vi "BenchA_v09_97.vi"() -> ()   [LabVIEW 2017]
uses:
  x64/Debug/BERTTA.dll
panel:
  out "element":bool
  out "Started:":string
  in  "SHUTDOWN":bool
  in  "MASTER CONTROL":bool
  in  "Tab Control":T1(tab)
  out "Output File":path caption="selected path"
  in  "Browse folder":path=path "" caption="start path"
  in  "Read Seq":bool
  in  "Save Seq":bool
  in  "Configuration file":path=path "C:/Users/shresplab/Desktop/BerttaConfiguration.lvm" caption="Filename"
  in  "OK Button 2":bool
  out "Boolean":bool
  in  "User (initials)":string
  in  "Project name":string
  in  "Description":string
  out "PUMP1":bool
  out "Target amount":dbl
  out "Scale weight":dbl
  out "Amount now":dbl
  out "Flow rate":dbl
  out "Time to target":dbl format="%<%H:%M:%S>t"
  out "Current step":dbl
  out "Target":dbl
  out "Amount now":dbl
  out "Amount now":dbl
  out "Target":dbl
  out "Current step":dbl
  out "Time to target":dbl format="%<%H:%M:%S>t"
  out "Flow rate":dbl
  out "Amount now":dbl
  out "Scale weight":dbl
  out "Target amount":dbl
  out "PUMP2":bool
  out "Sensor OK 6":bool
  out "Sensor OK 5":bool
  out "Sensor OK 4":bool
  out "Sensor OK 3":bool
  in  "OK Button":bool
  in  "Add comment":string
  out "PUMP3":bool
  out "Target amount":dbl
  out "Scale weight":dbl
  out "Amount now":dbl
  out "Flow rate":dbl
  out "Time to target":dbl format="%<%H:%M:%S>t"
  out "Current step":dbl
  out "Target":dbl
  out "Amount now":dbl
  out "Tr":dbl
  out "Tj in":dbl
  out "Tj out":dbl
  out "T set":dbl
  out "Current step":i32
  out "RPM":dbl
  out "Torque 2":dbl
  out "Waveform Chart 5":dynamicdata(graph)
  out "Waveform Chart 6":dynamicdata(graph)
  out "Waveform Chart 7":dynamicdata(graph)
  in  "Tab Control 2":T2(tab)
  out "Waveform Chart 3":dynamicdata(graph)
  out "Waveform Chart 8":dynamicdata(graph)
  out "Waveform Chart 11":dynamicdata(graph)
  out "Waveform Chart 13":dynamicdata(graph)
  out "Waveform Chart 9":dynamicdata(graph)
  out "Table":string[][](table)=[["14.8.2017 18.06.59", "0,000000", "417,670000", "-0,150000", "1,000000", "22,220000", "23,366837", "23,574959", "23,985852", "23,690000", "240,000000", "4,000000", "0,000000", "397,000000", "-397,000000", "1,000000"], ["14.8.2017 18.07.06", "0,000000", "417,640000", "-0,120000", "1,000000", "22,220000", "23,763115", "23,906257", "23,985694", "23,680000", "240,000000", "4,000000", "0,000000", "397,000000", "-397,000000", "1,000000"], ["14.8.2017 18.07.13", "0,000000", "417,640000", "-0,120000", "1,000000", "22,220000", "23,965922", "24,013440", "23,984906", "23,670000", "240,000000", "4,100000", "3,000000", "397,000000", "-397,000000", "1,000000"], ["14.8.2017 18.07.21", "0,000000", "417,640000", "-0,120000", "1,000000", "22,220000", "23,943860", "23,900110", "23,987113", "23,670000", "240,000000", "4,000000", "0,000000", "397,000000", "-397,000000", "1,000000"], ["14.8.2017 18.07.28", "0,000000", "417,640000", "-0,120000", "1,000000", "22,220000", "23,736328", "23,600018", "23,989004", "23,660000", "240,000000", "4,000000", "0,000000", "397,000000", "-397,000000", "1,000000"], ["14.8.2017 18.07.36", "0,000000", "417,640000", "-0,120000", "1,000000", "22,220000", "23,480910", "23,324538", "23,991053", "23,660000", "240,000000", "4,000000", "0,000000", "397,000000", "-397,000000", "1,000000"], ["14.8.2017 18.07.43", "0,000000", "417,640000", "-0,120000", "2,000000", "22,220000", "23,195579", "23,008270", "23,999093", "23,650000", "240,000000", "4,000000", "0,000000", "397,000000", "-397,000000", "1,000000"], ["14.8.2017 18.07.51", "0,000000", "417,650000", "-417,650000", "1,000000", "22,220000", "22,862541", "22,649021", "24,003979", "23,650000", "240,000000", "4,000000", "0,000000", "397,000000", "-397,000000", "2,000000"], ["14.8.2017 18.07.58", "0,000000", "417,640000", "0,010000", "1,000000", "22,220000", "22,541353", "22,354878", "24,005398", "23,650000", "240,000000", "4,000000", "0,000000", "397,000000", "-397,000000", "1,000000"], ["14.8.2017 18.08.06", "0,000000", "417,640000", "0,010000", "1,000000", "22,220000", "22,347931", "22,253738", "24,007605", "23,640000", "240,000000", "4,100000", "0,000000", "397,000000", "-397,000000", "1,000000"], ["14.8.2017 18.08.13", "0,000000", "417,640000", "0,010000", "1,000000", "22,220000", "22,329030", "22,302102", "24,006028", "23,640000", "240,000000", "4,000000", "0,000000", "395,820000", "-395,820000", "1,000000"], ["14.8.2017 18.08.20", "0,000000", "417,640000", "0,010000", "1,000000", "22,220000", "22,466849", "22,511320", "24,002403", "23,630000", "240,000000", "4,000000", "0,000000", "395,830000", "-0,010000", "1,000000"], ["14.8.2017 18.08.28", "0,000000", "417,640000", "0,010000", "1,000000", "22,220000", "22,707062", "22,835101", "24,000984", "23,620000", "240,000000", "4,000000", "0,000000", "395,830000", "-0,010000", "1,000000"], ["14.8.2017 18.08.35", "0,000000", "417,640000", "0,010000", "1,000000", "22,220000", "23,054104", "23,232979", "24,001299", "23,600000", "240,000000", "4,000000", "0,000000", "395,830000", "-0,010000", "1,000000"], ["14.8.2017 18.08.43", "0,000000", "417,640000", "0,010000", "1,000000", "22,220000", "23,412371", "23,522793", "24,002560", "23,590000", "240,000000", "4,000000", "0,000000", "395,820000", "0,000000", "1,000000"], ["14.8.2017 18.08.51", "0,000000", "417,640000", "0,010000", "1,000000", "22,220000", "23,596247", "23,656125", "24,003821", "23,580000", "240,000000", "4,000000", "0,000000", "395,820000", "0,000000", "1,000000"]]
  out "Boolean 4":bool
  out "Boolean 3":bool
  out "Boolean 2":bool
  in  "Reset 6":bool
  in  "Manual/Ramp":bool=TRUE
  in  "Array":dbl[][](array[numeric])=[[20.0, 0.0], [20.0, 0.0], [20.0, 0.0]]
  in  "?":bool
  in  "Time":dbl format="Time to target (min):                %#_g"
  out "Current temp":dbl format="Current temperature (S1):   %#_6g"
  in  "OK Button 3":bool
  in  "T ext / T ext 2":enum32{"Sensor 1", "Sensor 2"}(radio)
  out "Sensor OK":bool
  in  "T fail":dbl=20.0 format="Failsafe temperature:              %#_g"
  in  "Setpoint":dbl=20.0 format="Temperature target:                %#_6g"
  in  "Manual select":T3(radio)
  out "Waveform Chart":dynamicdata(graph)
  out "T external 2":dbl format="Current temperature (S2):    %#_g"
  in  "UPDATE TEMP":bool
  out "Led11 5":bool
  out "RPM":dbl format="%_4f"
  out "Led10 3":bool
  out "Led9 3":bool
  out "Led8 3":bool
  out "Led7 3":bool
  out "Led6 3":bool
  out "Led5 3":bool
  out "Led4 3":bool
  out "Led3 3":bool
  out "Led2 3":bool
  out "Led1 3":bool
  in  "PumpSeq 4":dbl[][](array[numeric])=[[0.0, 0.0, 0.0, 0.0, 0.0, 0.0, 0.0, 0.0, 0.0, 0.0], [0.0, 0.0, 0.0, 0.0, 0.0, 0.0, 0.0, 0.0, 0.0, 0.0], [0.0, 0.0, 0.0, 0.0, 0.0, 0.0, 0.0, 0.0, 0.0, 0.0], [0.0, 0.0, 0.0, 0.0, 0.0, 0.0, 0.0, 0.0, 0.0, 0.0], [0.0, 0.0, 0.0, 0.0, 0.0, 0.0, 0.0, 0.0, 0.0, 0.0], [0.0, 0.0, 0.0, 0.0, 0.0, 0.0, 0.0, 0.0, 0.0, 0.0], [0.0, 0.0, 0.0, 0.0, 0.0, 0.0, 0.0, 0.0, 0.0, 0.0], [0.0, 0.0, 0.0, 0.0, 0.0, 0.0, 0.0, 0.0, 0.0, 0.0], [0.0, 0.0, 0.0, 0.0, 0.0, 0.0, 0.0, 0.0, 0.0, 0.0], [0.0, 0.0, 0.0, 0.0, 0.0, 0.0, 0.0, 0.0, 0.0, 0.0]]
  in  "?":bool
  out "Flow rate (g/min)":dbl
  out "Scale reading":dbl
  out "Step amount now":dbl
  in  "Grams / min":dbl
  out "Waveform Chart 14":dynamicdata(graph)
  in  "?":bool
  out "Total amount now":dbl
  out "Led11 4":bool
  in  "Reset 5":bool
  out "Elapsed / step":i32
  out "Time to target":dbl format="%<%H:%M:%S>t"
  in  "OK Button 4":bool
  out "Led11":bool
  out "RPM":dbl format="%_4f"
  out "Led10":bool
  out "Led9":bool
  out "Led8":bool
  out "Led7":bool
  out "Led6":bool
  out "Led5":bool
  out "Led4":bool
  out "Led3":bool
  out "Led2":bool
  out "Led1":bool
  in  "PumpSeq 2":dbl[][](array[numeric])=[[0.0, 0.0, 0.0, 0.0, 0.0, 0.0, 0.0, 0.0, 0.0, 0.0], [0.0, 0.0, 0.0, 0.0, 0.0, 0.0, 0.0, 0.0, 0.0, 0.0], [0.0, 0.0, 0.0, 0.0, 0.0, 0.0, 0.0, 0.0, 0.0, 0.0], [0.0, 0.0, 0.0, 0.0, 0.0, 0.0, 0.0, 0.0, 0.0, 0.0], [0.0, 0.0, 0.0, 0.0, 0.0, 0.0, 0.0, 0.0, 0.0, 0.0], [0.0, 0.0, 0.0, 0.0, 0.0, 0.0, 0.0, 0.0, 0.0, 0.0], [0.0, 0.0, 0.0, 0.0, 0.0, 0.0, 0.0, 0.0, 0.0, 0.0], [0.0, 0.0, 0.0, 0.0, 0.0, 0.0, 0.0, 0.0, 0.0, 0.0], [0.0, 0.0, 0.0, 0.0, 0.0, 0.0, 0.0, 0.0, 0.0, 0.0], [0.0, 0.0, 0.0, 0.0, 0.0, 0.0, 0.0, 0.0, 0.0, 0.0]]
  in  "?":bool
  out "Flow rate (g/min)":dbl
  out "Scale reading":dbl
  out "Step amount now":dbl
  in  "Grams / min":dbl
  out "Waveform Chart 10":dynamicdata(graph)
  in  "?":bool
  out "Total amount now":dbl
  out "Led11":bool
  in  "Reset 3":bool
  out "Elapsed / step":i32
  out "Time to target":dbl format="%<%H:%M:%S>t"
  in  "OK Button 5":bool
  out "Led11 3":bool
  out "RPM":dbl format="%_4f"
  out "Led10 2":bool
  out "Led9 2":bool
  out "Led8 2":bool
  out "Led7 2":bool
  out "Led6 2":bool
  out "Led5 2":bool
  out "Led4 2":bool
  out "Led3 2":bool
  out "Led2 2":bool
  out "Led1 2":bool
  in  "PumpSeq 3":dbl[][](array[numeric])=[[0.0, 0.0, 0.0, 0.0, 0.0, 0.0, 0.0, 0.0, 0.0, 0.0], [0.0, 0.0, 0.0, 0.0, 0.0, 0.0, 0.0, 0.0, 0.0, 0.0], [0.0, 0.0, 0.0, 0.0, 0.0, 0.0, 0.0, 0.0, 0.0, 0.0], [0.0, 0.0, 0.0, 0.0, 0.0, 0.0, 0.0, 0.0, 0.0, 0.0], [0.0, 0.0, 0.0, 0.0, 0.0, 0.0, 0.0, 0.0, 0.0, 0.0], [0.0, 0.0, 0.0, 0.0, 0.0, 0.0, 0.0, 0.0, 0.0, 0.0], [0.0, 0.0, 0.0, 0.0, 0.0, 0.0, 0.0, 0.0, 0.0, 0.0], [0.0, 0.0, 0.0, 0.0, 0.0, 0.0, 0.0, 0.0, 0.0, 0.0], [0.0, 0.0, 0.0, 0.0, 0.0, 0.0, 0.0, 0.0, 0.0, 0.0], [0.0, 0.0, 0.0, 0.0, 0.0, 0.0, 0.0, 0.0, 0.0, 0.0]]
  in  "?":bool
  out "Flow rate (g/min)":dbl
  out "Scale reading":dbl
  out "Step amount now":dbl
  in  "Grams / min":dbl
  out "Waveform Chart 12":dynamicdata(graph)
  in  "?":bool
  out "Total amount now":dbl
  out "Led11 2":bool
  in  "Reset 4":bool
  out "Elapsed / step":i32
  out "Time to target":dbl format="%<%H:%M:%S>t"
  in  "OK Button 6":bool
  in  "Remote / Manual":bool
  in  "Set RPM":i32
  out "RPM":dbl
  out "Torque":dbl
  out "Waveform Chart 4":dynamicdata(graph)
  in  "OK Button 7":bool
  out "PortDev out":dbl[](array[numeric])
  in  "Save PortDev":bool
  out "PortDev in":dbl[](array[numeric])
  in  "dev1":i32
  in  "dev2":i32
  in  "dev3":i32
  in  "dev4":i32
  in  "dev5":i32
  in  "dev6":i32
  in  "dev8":i32
  in  "port1":i32
  in  "port2":i32
  in  "port3":i32
  in  "port4":i32
  in  "port5":i32
  in  "port6":i32
  in  "port7":i32
  in  "port8":i32
  in  "dev7":i32
  in  "Treshold (T/C)":dbl=0.5
  out "DAQ 9217 (PT100)":errorcluster
  out "Config File":dbl[][](array[numeric])
  # "Temperature sensor:"
  # "Manual control:"
  # "PUMP & SCALE 1"
  # "STEP"
  # "TOTAL"
  # "PUMP & SCALE 2"
  # "STEP"
  # "TOTAL"
  # "PUMP & SCALE 3"
  # "STEP"
  # "TOTAL"
  # "Temperature control parameter"
  # "Secondary temperature sensor"
  # "Temp target"
  # "Time target"
  # "Grams    /   min"
  # "End of sequence"
  # "Manual control"
  # "Grams    /   min"
  # "End of sequence"
  # "Manual control"
  # "Grams    /   min"
  # "End of sequence"
  # "Manual control"
  # "dev1 and dev2 always to port1 and 2\nport1 = port2 = Lauda\n\ndev3 and dev4 always to port3 and port4\nport3 = port4 = Heidolph"
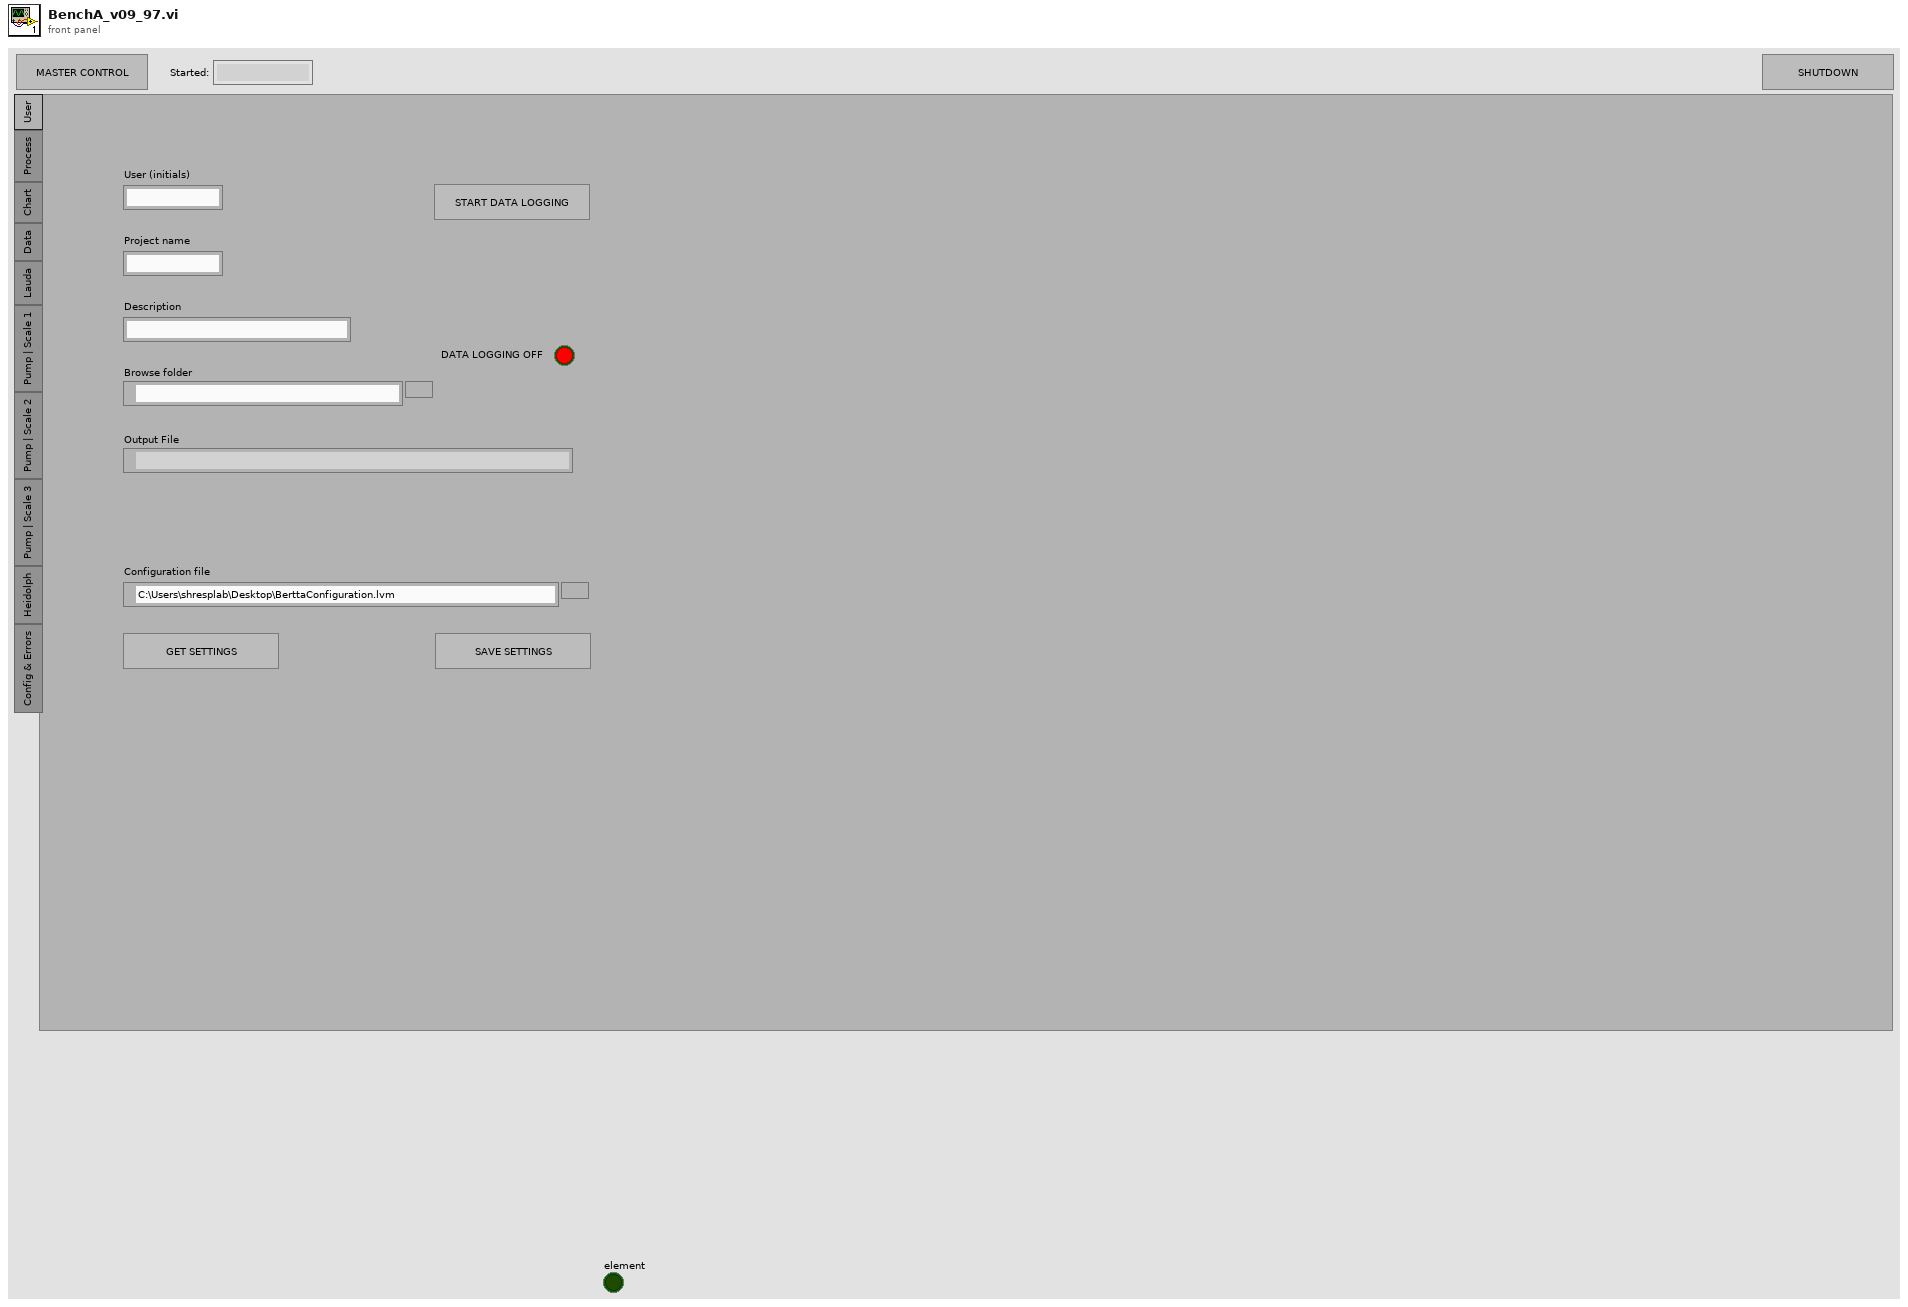
[diagram p1: front panel]
types:
  T1 = enum32{"User", "Process", "Chart", "Data", "Lauda", "Pump | Scale 1", "Pump | Scale 2", "Pump | Scale 3", "Heidolph", "Config & Errors"}
  T2 = enum32{"Temperatures", "Scale / Pump 1", "Scale / Pump 2", "Scale / Pump 3", "RPM / torque"}
  T3 = enum32{"Reactor temperature", "Jacket temperature"}
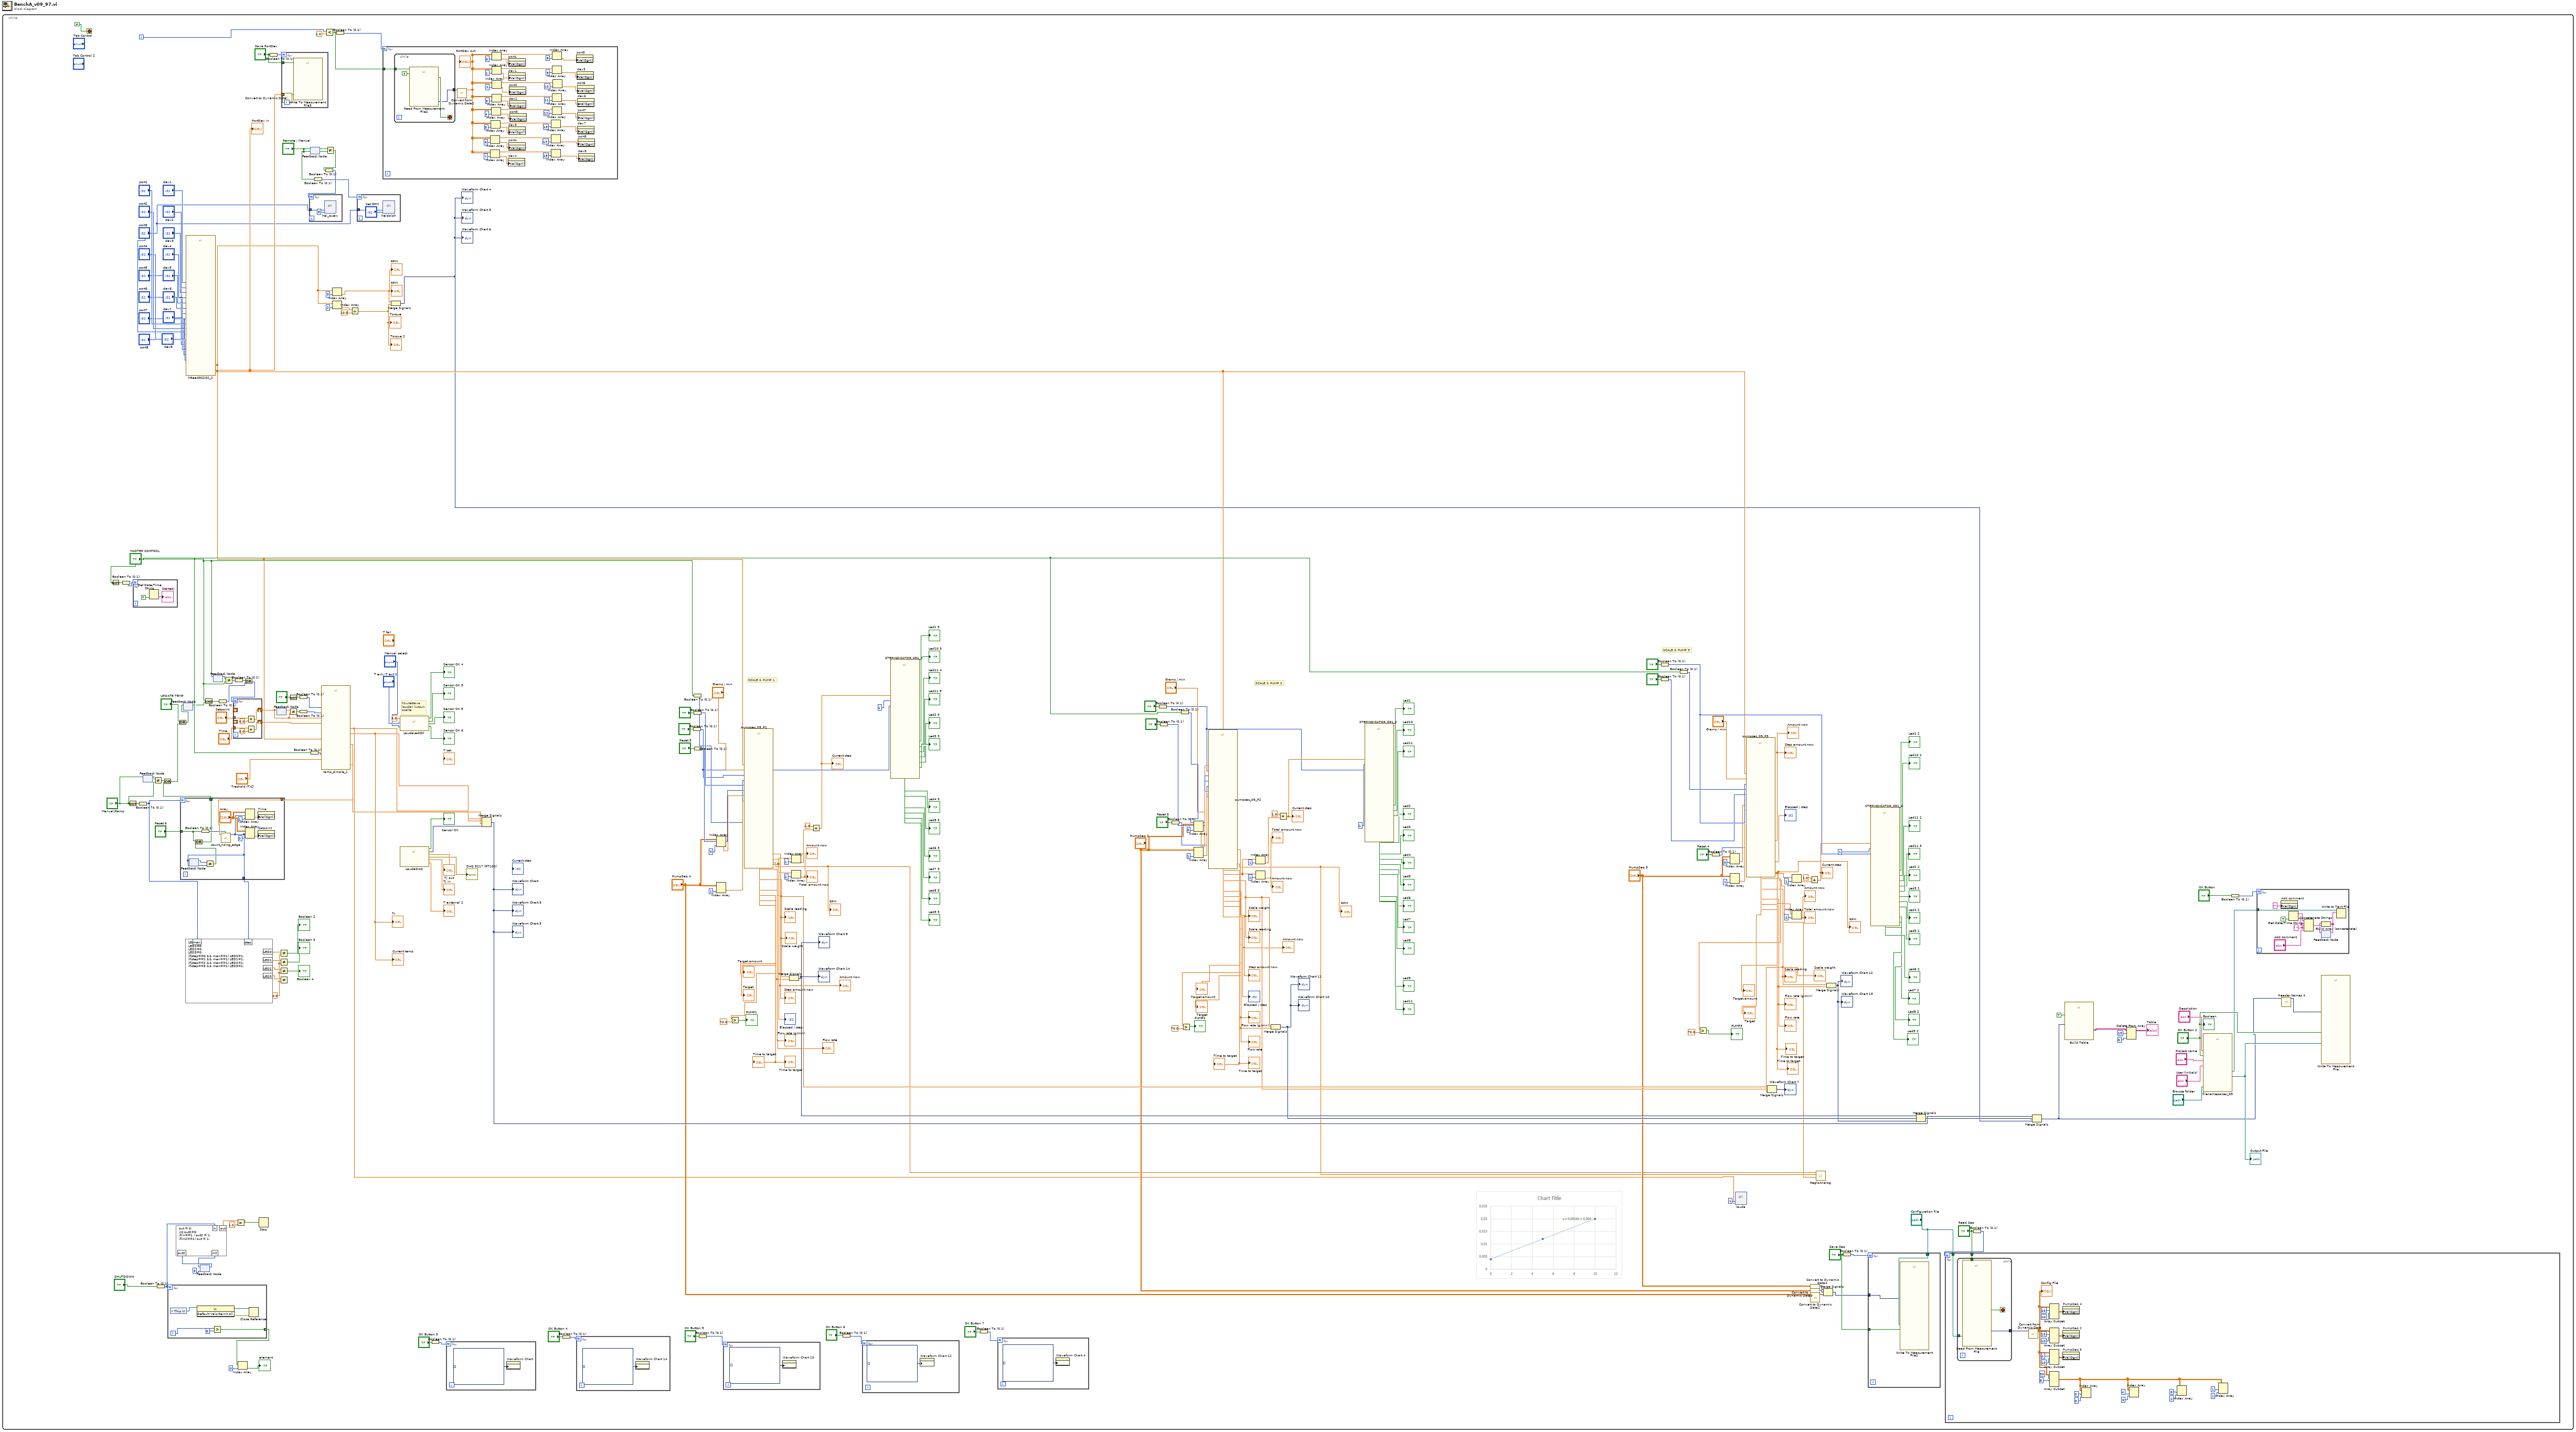
[diagram p0: block diagram]
diagram:
  n1 = while {
    i -> [w47]
    stop <- FALSE stop-if-true
    w33 = 0.0 ("y")
    # "Muutettava\nlaudan kutsun \nosalta"
    # "SCALE & PUMP 1"
    # "SCALE & PUMP 3"
    # "SCALE & PUMP 2"
    n2 = Not(x="MASTER CONTROL") -> (.not. x?=w275:bool)
    n3 = Boolean To (0,1)(Boolean=w275) -> (0, 1=w276:i16)
    n4 = Not(x="Manual/Ramp") -> (.not. x?=w40:bool)
    n5 = for {
      N: w276 -> [_]
      n6 = Get Date/Time String(want seconds? (F)=TRUE) -> (time string=→"Started:":string)  [unwired: 2 in, 1 out]
    }
    n7 = Boolean To (0,1)(Boolean=w40) -> (0, 1=w22:i16)
    n8 = feedback #1() -> (w28:bool)  [unwired: 1 in]
    n9 = feedback-in #1("Manual/Ramp") -> ()
    n10 = Not Equal?(x=w28, y="Manual/Ramp") -> (x != y?=w25:bool)
    n11 = Boolean To (0,1)(Boolean="SHUTDOWN") -> (0, 1=w260:i16)
    n12 = for {
      N: w260 -> [_]
      tunnel: [w391] -> w274 mode=indexing
      i -> [w393]
      n13 = control-ref of="This VI"() -> (w396:refnum<vi>)
      n14 = invoke class="VI" method="Default Vals.Reinit All"(reference=w396) -> (reference out=w394:refnum<vi>, error out=w395:errorcluster)  [unwired: 2 in, 1 out]
      n15 = Greater?(x=w393, y=0) -> (0:w391:bool)
      n16 = Close Reference(reference=w394, error in (no error)=w395) -> ()  [unwired: 1 out]
    }
    n17 = feedback #2() -> (w20:bool)  [unwired: 1 in]
    n18 = call "MReadRS232_2.vi"("port1"="port1", "dev1"="dev1", "port2"="port2", "dev2"="dev2", "port3"="port3", "dev7"="dev7", "dev8"="dev8", "port7"="port7", "port8"="port8", "dev5"="dev5", "port5"="port5", "dev4"="dev4", "dev6"="dev6", "port6"="port6", "port4"="port4", "dev3"="dev3") -> ("output array"=w51:dbl[], "params"=w12:dbl[])  [unwired: 2 in]
    "PortDev in" <- w51
    n19 = feedback #3(0) -> (w258:i32)
    n20 = formula code="out = 0;\nint out2=0;\nif(in==1 ) out2 = 1;\nif(in2==1) out = 1;"("in"=w260, "in2"=w258) -> ("out"=w262:dbl, "out2"=w259:i32)
    n21 = feedback-in #3(w259) -> ()
    n22 = And(x="MASTER CONTROL", y=w20) -> (x .and. y?=w80:bool)
    n23 = feedback #4() -> (w71:bool)  [unwired: 1 in]
    n24 = feedback-in #4("MASTER CONTROL") -> ()
    n25 = Boolean To (0,1)(Boolean=w80) -> (0, 1=w68:i16)
    n26 = Not Equal?(x=w71, y="MASTER CONTROL") -> (x != y?=w70:bool)
    n27 = Boolean To (0,1)(Boolean=w70) -> (0, 1=w67:i16)
    n28 = Equal?(x=w262, y=1.0) -> (x = y?=w261:bool)
    n29 = Index Array(array=w274, index=0) -> (element=→"element":bool)
    n30 = Or(x=w67, y=w68) -> (x .or. y?=w66:i16)
    n31 = for {
      N: w66 -> [_]
      tunnel: "Time" -> [w343]
      shift-right: [w342] -> w81
      shift-left: _ -> [_]
      tunnel: "Setpoint" -> [w340]
      shift-right: [w339] -> w78
      shift-left: _ -> [_]
      n32 = Add(x=w340, y=0.0) -> (x+y=w339:dbl)
      n33 = Add(x=w343, y=0.0) -> (x+y=w342:dbl)
    }
    n34 = Stop(stop? (T)=w261) -> ()
    n35 = Boolean To (0,1)(Boolean="Save PortDev") -> (0, 1=w50:i16)
    n36 = feedback-in #5(w78) -> ()
    n37 = feedback #5() -> (w79:dbl)  [unwired: 1 in]
    n38 = for {
      N: w50 -> [_]
      tunnel: w51 -> [w338]
      tunnel: "Save PortDev" -> [w336]
      n39 = call "Convert to Dynamic Data"("Array"=w338) -> ("Dynamic Data Type"=w337:dynamicdata)  [unwired: 3 in]
      n40 = call "Write To Measurement File3"("Signals"=w337, "Reset"=w336) -> ()  [unwired: 15 in, 3 out]
    }
    n41 = Not(x="?") -> (.not. x?=w74:bool)
    n42 = Not Equal?(x=w79, y=w78) -> (x != y?=w77:bool)
    n43 = Boolean To (0,1)(Boolean=w74) -> (0, 1=w76:i16)
    n44 = Boolean To (0,1)(Boolean=w77) -> (0, 1=w72:i16)
    n45 = Boolean To (0,1)(Boolean="MASTER CONTROL") -> (0, 1=w73:i16)
    n46 = feedback-in #6("Remote / Manual") -> ()
    n47 = feedback #6() -> (w17:bool)  [unwired: 1 in]
    n48 = Boolean To (0,1)(Boolean="Remote / Manual") -> (0, 1=w15:i16)
    n49 = call "ramp_simple_1.vi"("array"=w12, "treshold"="Treshold (T/C)", "time_set"=w81, "T_sp"=w78, "master"=w73, "reset"=w72, "pause"=w76) -> ("T control"=w1:dbl, "Tr"=w85:dbl, "Tin"=w84:dbl, "target_reached"=w38:dbl)  [unwired: 1 out]
    "Tr" <- w85
    "Current temp" <- w85
    n50 = for {
      N: w22 -> [_]
      tunnel: w38 -> [w295]
      tunnel: [w285] -> w26
      tunnel: "Reset 6" -> [w287]
      tunnel: [w288] -> w29
      n51 = feedback #7() -> (w289:i32)  [unwired: 1 in]
      n52 = Boolean To (0,1)(Boolean=w287) -> (0, 1=w290:i16)
      n53 = call "count_rising_edge.vi"("reset"=w290, "target_reached"=w295) -> ("element 2"=w288:i32)  [unwired: 9 in]
      n54 = feedback-in #7(w288) -> ()
      n55 = Not Equal?(x=w289, y=w288) -> (x != y?=w286:bool)
      n56 = Or(x=w287, y=w286) -> (x .or. y?=w285:bool)
      n57 = Index Array(array="Array", index (row)=w288, index (col)=1 ("disabled index (col)")) -> (element=w291:dbl)
      n58 = Index Array(array="Array", index (row)=w288, index (col)=0 ("disabled index (col)")) -> (element=w292:dbl)
      n59 = property on="Time" class="DigNum (strict)"("Val(Sgnl)"=w291) -> ()  [unwired: 2 in, 2 out]
      n60 = property on="Setpoint" class="DigNum (strict)"("Val(Sgnl)"=w292) -> ()  [unwired: 2 in, 2 out]
    }
    n61 = Or(x=w25, y=w26) -> (x .or. y?=w24:bool)
    n62 = Or(x="UPDATE TEMP", y=w24) -> (x .or. y?=w21:bool)
    n63 = feedback-in #2(w21) -> ()
    n64 = formula code="LED0=0;\nLED1=0;\nLED2=0;\nLED3=0;\nif(step==0 && man==1) LED0=1;\nif(step==1 && man==1) LED1=1;\nif(step==2 && man==1) LED2=1;\nif(step==3 && man==1) LED3=1;"("step"=w29, "man"=w22) -> ("LED0"=w37:dbl, "LED1"=w36:dbl, "LED2"=w35:dbl, "LED3"=w34:dbl)
    n65 = Not Equal?(x=w37, y=w33) -> (x != y?=→"Boolean 2":bool)
    n66 = Not Equal?(x=w36, y=w33) -> (x != y?=→"Boolean 3":bool)
    n67 = Not Equal?(x=w35, y=w33) -> (x != y?=→"Boolean 4":bool)
    n68 = Not Equal?(x=w34, y=w33) -> ()  [unwired: 1 out]
    n69 = Less?(x=w47, y=1.0) -> (x < y?=w45:bool)
    n70 = Not Equal?(x=w17, y="Remote / Manual") -> (x != y?=w16:bool)
    n71 = Boolean To (0,1)(Boolean=w16) -> (0, 1=w18:i16)
    n72 = for {
      N: w18 -> [_]
      tunnel: "port3" -> [w283]
      n73 = dll-call lib="C:/Users/shresplab/OneDrive - Kemira Oyj/Documents/GitHub/Bertta/BERTTA/x64/Debug/BERTTA.dll" fn="hei_query"("port"=w283, "q"=5) -> ()  [unwired: 6 in, 2 out]
    }
    n74 = Index Array(array=w12, index=3) -> (element=w9:dbl)
    "RPM" <- w9
    "RPM" <- w9
    n75 = Index Array(array=w12, index=2) -> (element=w11:dbl)
    n76 = Boolean To (0,1)(Boolean=w45) -> (0, 1=w46:i16)
    n77 = Divide(x=w11, y=10.0) -> (x/y=w8:dbl)
    "Torque" <- w8
    "Torque 2" <- w8
    n78 = for {
      N: w15 -> [_]
      tunnel: "port3" -> [w281]
      n79 = dll-call lib="C:/Users/shresplab/OneDrive - Kemira Oyj/Documents/GitHub/Bertta/BERTTA/x64/Debug/BERTTA.dll" fn="heidolph"("port"=w281, "speed"="Set RPM") -> ()  [unwired: 6 in, 2 out]
    }
    n80 = for {
      N: w46 -> [_]
      tunnel: w45 -> [w331]
      n81 = while {
        tunnel: [w334] -> w330
        tunnel: w331 -> [w332]
        stop <- w335 stop-if-true
        n82 = call "Read From Measurement File2"("Enable"=TRUE, "Reset"=w332) -> ("Signals"=w334:dynamicdata, "EOF?"=w335:bool)  [unwired: 4 in, 4 out]
      }
      n83 = call "Convert from Dynamic Data2"("Dynamic Data Type"=w330) -> ("Array"=w313:dbl[])  [unwired: 3 in]
      "PortDev out" <- w313
      n84 = Index Array(array=w313, index=6) -> (element=w306:dbl)
      n85 = Index Array(array=w313, index=7) -> (element=w305:dbl)
      n86 = Index Array(array=w313, index=5) -> (element=w307:dbl)
      n87 = Index Array(array=w313, index=4) -> (element=w308:dbl)
      n88 = Index Array(array=w313, index=0) -> (element=w312:dbl)
      n89 = Index Array(array=w313, index=1) -> (element=w311:dbl)
      n90 = Index Array(array=w313, index=3) -> (element=w309:dbl)
      n91 = Index Array(array=w313, index=2) -> (element=w310:dbl)
      n92 = property on="dev4" class="DigNum (strict)"("Val(Sgnl)"=w305) -> ()  [unwired: 2 in, 2 out]
      n93 = property on="dev3" class="DigNum (strict)"("Val(Sgnl)"=w307) -> ()  [unwired: 2 in, 2 out]
      n94 = property on="port4" class="DigNum (strict)"("Val(Sgnl)"=w306) -> ()  [unwired: 2 in, 2 out]
      n95 = property on="port1" class="DigNum (strict)"("Val(Sgnl)"=w312) -> ()  [unwired: 2 in, 2 out]
      n96 = property on="dev1" class="DigNum (strict)"("Val(Sgnl)"=w311) -> ()  [unwired: 2 in, 2 out]
      n97 = property on="port2" class="DigNum (strict)"("Val(Sgnl)"=w310) -> ()  [unwired: 2 in, 2 out]
      n98 = property on="dev2" class="DigNum (strict)"("Val(Sgnl)"=w309) -> ()  [unwired: 2 in, 2 out]
      n99 = property on="port3" class="DigNum (strict)"("Val(Sgnl)"=w308) -> ()  [unwired: 2 in, 2 out]
      n100 = Index Array(array=w313, index=14) -> (element=w298:dbl)
      n101 = Index Array(array=w313, index=15) -> (element=w297:dbl)
      n102 = Index Array(array=w313, index=13) -> (element=w299:dbl)
      n103 = Index Array(array=w313, index=12) -> (element=w300:dbl)
      n104 = Index Array(array=w313, index=8) -> (element=w304:dbl)
      n105 = Index Array(array=w313, index=9) -> (element=w303:dbl)
      n106 = Index Array(array=w313, index=11) -> (element=w301:dbl)
      n107 = Index Array(array=w313, index=10) -> (element=w302:dbl)
      n108 = property on="port5" class="DigNum (strict)"("Val(Sgnl)"=w304) -> ()  [unwired: 2 in, 2 out]
      n109 = property on="dev5" class="DigNum (strict)"("Val(Sgnl)"=w303) -> ()  [unwired: 2 in, 2 out]
      n110 = property on="port6" class="DigNum (strict)"("Val(Sgnl)"=w302) -> ()  [unwired: 2 in, 2 out]
      n111 = property on="dev6" class="DigNum (strict)"("Val(Sgnl)"=w301) -> ()  [unwired: 2 in, 2 out]
      n112 = property on="port7" class="DigNum (strict)"("Val(Sgnl)"=w300) -> ()  [unwired: 2 in, 2 out]
      n113 = property on="dev7" class="DigNum (strict)"("Val(Sgnl)"=w299) -> ()  [unwired: 2 in, 2 out]
      n114 = property on="port8" class="DigNum (strict)"("Val(Sgnl)"=w298) -> ()  [unwired: 2 in, 2 out]
      n115 = property on="dev8" class="DigNum (strict)"("Val(Sgnl)"=w297) -> ()  [unwired: 2 in, 2 out]
    }
    n116 = Merge Signals(w9, w8) -> (w7:dynamicdata)
    "Waveform Chart 4" <- w7
    "Waveform Chart 6" <- w7
    "Waveform Chart 9" <- w7
    n117 = call "LaudaLedCtrl.vi"("Manual select"="Manual select", "T ext / T ext in"="T ext / T ext 2", "Lauda port"=9.0) -> ("Sensor OK 5"=→"Sensor OK 5":bool, "Sensor OK 3"=→"Sensor OK 3":bool, "Sensor OK 4"=→"Sensor OK 4":bool, "Sensor OK 6"=→"Sensor OK 6":bool)  [unwired: 5 in]
    n118 = call "LaudaDAQ.vi"() -> ("error out"=→"DAQ 9217 (PT100)":errorcluster, 1:"Tj out"=→"Tj out":dbl, "data"=w150:dynamicdata, "Sensor OK"=→"Sensor OK":bool, 4:"Tj out"=→"Tj in":dbl, "T external 2"=→"T external 2":dbl)  [unwired: 6 in]
    n119 = Boolean To (0,1)(Boolean="OK Button 3") -> (0, 1=w96:i16)
    n120 = for {
      N: w96 -> [_]
      n121 = property on="Waveform Chart" class="WFChart (strict)"("History Data"=dynamicdata[] []) -> ()  [unwired: 2 in, 2 out]
    }
    n122 = Merge Signals(w1, w85, w84, w150) -> (w151:dynamicdata)
    "Waveform Chart 3" <- w151
    "Waveform Chart" <- w151
    "Waveform Chart 5" <- w151
    n123 = Boolean To (0,1)(Boolean="OK Button 4") -> (0, 1=w94:i16)
    n124 = for {
      N: w94 -> [_]
      n125 = property on="Waveform Chart 14" class="WFChart (strict)"("History Data"=dynamicdata[] []) -> ()  [unwired: 2 in, 2 out]
    }
    n126 = Boolean To (0,1)(Boolean="?") -> (0, 1=w159:i16)
    n127 = Boolean To (0,1)(Boolean="?") -> (0, 1=w163:i16)
    n128 = Boolean To (0,1)(Boolean="MASTER CONTROL") -> (0, 1=w155:i16)
    n129 = Boolean To (0,1)(Boolean="Reset 5") -> (0, 1=w162:i16)
    n130 = Boolean To (0,1)(Boolean="OK Button 5") -> (0, 1=w92:i16)
    n131 = Index Array(array="PumpSeq 4", index (col)=0) -> (element=w167:dbl[])  [unwired: 1 in]
    n132 = Index Array(array="PumpSeq 4", index (col)=1) -> (element=w188:dbl[])  [unwired: 1 in]
    n133 = for {
      N: w92 -> [_]
      n134 = property on="Waveform Chart 10" class="WFChart (strict)"("History Data"=dynamicdata[] []) -> ()  [unwired: 2 in, 2 out]
    }
    n135 = call "pumpsec_09_P1.vi"("reset"=w162, "master"=w155, "manual"=w159, "pause"=w163, "Array"=w12, "Target"=w167, "fr_manual"="Grams / min", "Time"=w188) -> ("pumpCtrl"=w134:dbl, "totaltarget"=→"Target":dbl, "target_step"=→"Target amount":dbl, "REGLO D"=w5:dbl, "time_to_target"=→"Time to target" →"Time to target":dbl, "step_fr"=w111:dbl, "amount_step"=→"Amount now" →"Step amount now":dbl, "Scale"=w146:dbl, "elapsed_step"=→"Elapsed / step":dbl, "params"=w185:dbl[])  [unwired: 8 in, 2 out]
    "Flow rate" <- w111
    "Scale weight" <- w146
    "Scale reading" <- w146
    "Flow rate (g/min)" <- w111
    "RPM" <- w5
    n136 = Greater?(x=w134, y=70.0) -> (0:→"PUMP1":bool)
    n137 = Merge Signals(w146, w111) -> (w154:dynamicdata)
    "Waveform Chart 8" <- w154
    "Waveform Chart 14" <- w154
    n138 = Index Array(array=w185, index=1) -> (element=w182:dbl)
    n139 = Index Array(array=w185, index=2) -> (element=→"Amount now" →"Total amount now":dbl)
    n140 = Add(x=1.0, y=w182) -> (x+y=w112:dbl)
    "Current step" <- w112
    n141 = Boolean To (0,1)(Boolean="OK Button 6") -> (0, 1=w90:i16)
    n142 = for {
      N: w90 -> [_]
      n143 = property on="Waveform Chart 12" class="WFChart (strict)"("History Data"=dynamicdata[] []) -> ()  [unwired: 2 in, 2 out]
    }
    n144 = call "STEPINDICATOR_091_2.vi"("current step"=w112, "enable"=i16 1, "manual"=w159) -> ("Led 8"=→"Led8 3":bool, "Led 10"=→"Led10 3":bool, "Led 11"=→"Led11 4":bool, "Led 7"=→"Led7 3":bool, "Led 1"=→"Led1 3":bool, "Led 6"=→"Led6 3":bool, "Led 2"=→"Led2 3":bool, "Led 12"=→"Led11 5":bool, "Led 5"=→"Led5 3":bool, "Led 4"=→"Led4 3":bool, "Led 3"=→"Led3 3":bool, "Led 9"=→"Led9 3":bool)  [unwired: 1 in]
    n145 = Boolean To (0,1)(Boolean="OK Button 7") -> (0, 1=w88:i16)
    n146 = for {
      N: w88 -> [_]
      n147 = property on="Waveform Chart 4" class="WFChart (strict)"("History Data"=dynamicdata[] []) -> ()  [unwired: 2 in, 2 out]
    }
    n148 = Boolean To (0,1)(Boolean="?") -> (0, 1=w222:i16)
    n149 = Boolean To (0,1)(Boolean="?") -> (0, 1=w249:i16)
    n150 = Boolean To (0,1)(Boolean="Reset 3") -> (0, 1=w247:i16)
    n151 = Boolean To (0,1)(Boolean="MASTER CONTROL") -> (0, 1=w241:i16)
    n152 = Index Array(array="PumpSeq 2", index (col)=0 ("disabled index (col)")) -> (element=w252:dbl[])  [unwired: 1 in]
    n153 = Index Array(array="PumpSeq 2", index (col)=1 ("disabled index (col)")) -> (element=w251:dbl[])  [unwired: 1 in]
    n154 = call "pumpsec_09_P2.vi"("reset"=w247, "master"=w241, "manual"=w222, "pause"=w249, "Array"=w12, "Target"=w252, "fr_manual"="Grams / min", "Time"=w251) -> ("pumpCtrl"=w130:dbl, "totaltarget"=→"Target":dbl, "target_step"=→"Target amount":dbl, "REGLO D"=w4:dbl, "time_to_target"=→"Time to target" →"Time to target":dbl, "step_fr"=w149:dbl, "amount_step"=→"Amount now" →"Step amount now":dbl, "Scale"=w145:dbl, "elapsed_step"=→"Elapsed / step":dbl, "params"=w242:dbl[])  [unwired: 8 in, 2 out]
    "Scale weight" <- w145
    "Flow rate" <- w149
    "Scale reading" <- w145
    "Flow rate (g/min)" <- w149
    "RPM" <- w4
    n155 = Greater?(x=w130, y=70.0) -> (0:→"PUMP2":bool)
    n156 = Index Array(array=w242, index=1) -> (element=w245:dbl)
    n157 = Index Array(array=w242, index=2) -> (element=→"Amount now" →"Total amount now":dbl)
    n158 = Merge Signals(w145, w149) -> (w156:dynamicdata)
    "Waveform Chart 11" <- w156
    "Waveform Chart 10" <- w156
    n159 = Add(x=1.0, y=w245) -> (x+y=w239:dbl)
    "Current step" <- w239
    n160 = call "STEPINDICATOR_091_2.vi"("current step"=w239, "enable"=i16 1, "manual"=w222) -> ("Led 8"=→"Led8":bool, "Led 10"=→"Led10":bool, "Led 11"=→"Led11":bool, "Led 7"=→"Led7":bool, "Led 1"=→"Led1":bool, "Led 6"=→"Led6":bool, "Led 2"=→"Led2":bool, "Led 12"=→"Led11":bool, "Led 5"=→"Led5":bool, "Led 4"=→"Led4":bool, "Led 3"=→"Led3":bool, "Led 9"=→"Led9":bool)  [unwired: 1 in]
    n161 = Boolean To (0,1)(Boolean="?") -> (0, 1=w216:i16)
    n162 = Boolean To (0,1)(Boolean="?") -> (0, 1=w215:i16)
    n163 = Boolean To (0,1)(Boolean="MASTER CONTROL") -> (0, 1=w217:i16)
    n164 = Boolean To (0,1)(Boolean="Reset 4") -> (0, 1=w197:i16)
    n165 = Index Array(array="PumpSeq 3", index (col)=0 ("disabled index (col)")) -> (element=w200:dbl[])  [unwired: 1 in]
    n166 = Index Array(array="PumpSeq 3", index (col)=1 ("disabled index (col)")) -> (element=w199:dbl[])  [unwired: 1 in]
    n167 = dll-call lib="C:/Users/shresplab/OneDrive - Kemira Oyj/Documents/GitHub/Bertta/BERTTA/x64/Debug/BERTTA.dll" fn="lauda"("port"=1, "set_temp"=w1) -> ()  [unwired: 6 in, 2 out]
    n168 = call "pumpsec_09_P3.vi"("reset"=w197, "master"=w217, "manual"=w216, "pause"=w215, "Array"=w12, "Target"=w200, "fr_manual"="Grams / min", "Time"=w199) -> ("pumpCtrl"=w127:dbl, "totaltarget"=→"Target":dbl, "target_step"=→"Target amount":dbl, "REGLO D"=w3:dbl, "time_to_target"=→"Time to target" →"Time to target":dbl, "step_fr"=w148:dbl, "amount_step"=→"Amount now" →"Step amount now":dbl, "Scale"=w144:dbl, "elapsed_step"=→"Elapsed / step":dbl, "params"=w190:dbl[])  [unwired: 8 in, 2 out]
    "Scale weight" <- w144
    "Flow rate" <- w148
    "Scale reading" <- w144
    "Flow rate (g/min)" <- w148
    "RPM" <- w3
    n169 = Greater?(x=w127, y=70.0) -> (0:→"PUMP3":bool)
    n170 = Merge Signals(w146, w145, w144) -> (→"Waveform Chart 7":dynamicdata)
    n171 = Index Array(array=w190, index=1) -> (element=w191:dbl)
    n172 = Index Array(array=w190, index=2) -> (element=→"Amount now" →"Total amount now":dbl)
    n173 = Add(x=1.0, y=w191) -> (x+y=w189:dbl)
    "Current step" <- w189
    n174 = call "Convert to Dynamic Data4"("2D Array"="PumpSeq 3") -> ("Dynamic Data Type"=w103:dynamicdata)  [unwired: 3 in]
    n175 = call "Convert to Dynamic Data3"("2D Array"="PumpSeq 2") -> ("Dynamic Data Type"=w105:dynamicdata)  [unwired: 3 in]
    n176 = call "Convert to Dynamic Data2"("2D Array"="PumpSeq 4") -> ("Dynamic Data Type"=w108:dynamicdata)  [unwired: 3 in]
    n177 = call "RegloAnalog.vi"("REGLO D"=w3, "REGLO D 2"=w4, "REGLO D 3"=w5) -> ()  [unwired: 9 in]
    n178 = Merge Signals(w103, w105, w108) -> (w107:dynamicdata)
    n179 = Merge Signals(w144, w148) -> (w153:dynamicdata)
    "Waveform Chart 13" <- w153
    "Waveform Chart 12" <- w153
    n180 = Boolean To (0,1)(Boolean="Save Seq") -> (0, 1=w102:i16)
    n181 = for {
      N: w102 -> [_]
      tunnel: w107 -> [w389]
      tunnel: "Configuration file" -> [w390]
      tunnel: "Save Seq" -> [w388]
      n182 = call "Write To Measurement File2"("Signals"=w389, "Reset"=w388, "Filename"=w390) -> ()  [unwired: 14 in, 3 out]
    }
    n183 = call "STEPINDICATOR_091_4.vi"("current step"=w189, "enable"=i16 1, "manual"=w216) -> ("Led 8"=→"Led8 2":bool, "Led 10"=→"Led10 2":bool, "Led 11"=→"Led11 2":bool, "Led 7"=→"Led7 2":bool, "Led 1"=→"Led1 2":bool, "Led 6"=→"Led6 2":bool, "Led 2"=→"Led2 2":bool, "Led 12"=→"Led11 3":bool, "Led 5"=→"Led5 2":bool, "Led 4"=→"Led4 2":bool, "Led 3"=→"Led3 2":bool, "Led 9"=→"Led9 2":bool)  [unwired: 1 in]
    n184 = Merge Signals(w154, w156, w153) -> (w152:dynamicdata)
    n185 = Boolean To (0,1)(Boolean="Read Seq") -> (0, 1=w101:i16)
    n186 = for {
      N: w101 -> [_]
      tunnel: "Configuration file" -> [w361]
      tunnel: "Read Seq" -> [w360]
      n187 = while {
        tunnel: [w387] -> w383
        tunnel: w361 -> [w386]
        tunnel: w360 -> [w384]
        stop <- w385 stop-if-true
        n188 = call "Read From Measurement File"("Filename"=w386, "Reset"=w384) -> ("Signals"=w387:dynamicdata, "EOF?"=w385:bool)  [unwired: 4 in, 4 out]
      }
      n189 = call "Convert from Dynamic Data"("Dynamic Data Type"=w383) -> ("Array"=w373:dbl[][])  [unwired: 3 in]
      "Config File" <- w373
      n190 = Array Subset(array=w373, index (row)=20 ("index"), length (row)=10 ("length")) -> (w380:dbl[][])  [unwired: 2 in]
      n191 = Array Subset(array=w373, index (row)=10 ("index"), length (row)=10 ("length")) -> (w375:dbl[][])  [unwired: 2 in]
      n192 = Array Subset(array=w373, index (row)=0 ("index"), length (row)=10 ("length")) -> (w374:dbl[][])  [unwired: 2 in]
      n193 = Array Subset(array=w373, index (row)=30 ("index"), length (row)=8 ("length")) -> (w362:dbl[][])  [unwired: 2 in]
      n194 = property on="PumpSeq 4" class="Arr (strict)"("Val(Sgnl)"=w380) -> ()  [unwired: 2 in, 2 out]
      n195 = property on="PumpSeq 2" class="Arr (strict)"("Val(Sgnl)"=w375) -> ()  [unwired: 2 in, 2 out]
      n196 = property on="PumpSeq 3" class="Arr (strict)"("Val(Sgnl)"=w374) -> ()  [unwired: 2 in, 2 out]
      n197 = Index Array(array=w362, index (row)=2, index (col)=0 ("disabled index (col)")) -> ()  [unwired: 1 out]
      n198 = Index Array(array=w362, index (row)=4, index (col)=0 ("disabled index (col)")) -> ()  [unwired: 1 out]
      n199 = Index Array(array=w362, index (row)=0, index (col)=1 ("disabled index (col)")) -> ()  [unwired: 1 out]
      n200 = Index Array(array=w362, index (row)=1, index (col)=1 ("disabled index (col)")) -> ()  [unwired: 1 out]
    }
    n201 = Merge Signals(w151, w152, w7) -> (w43:dynamicdata)
    n202 = call "Build Table"("Include time data"=TRUE, "Signals"=w43) -> ("Table"=w270:string[][])  [unwired: 3 in, 6 out]
    n203 = Delete From Array(array=w270, length=13, index (col)=0 ("index (row)")) -> (array with subset deleted=→"Table":string[][])  [unwired: 1 in, 1 out]
    n204 = call "filenameparser_09.vi"("Description"="Description", "start path"="Browse folder", "Project name"="Project name", "User (initials)"="User (initials)", "OK Button in"="OK Button 2") -> ("appended path 2"=w86:path, "appended path"=w266:path)  [unwired: 4 in, 1 out]
    "Output File" <- w86
    n205 = Boolean To (0,1)(Boolean="OK Button") -> (0, 1=w265:i16)
    n206 = for {
      N: w265 -> [_]
      tunnel: w266 -> [w352]
      w356 = " " ("string")
      n207 = property on="Add comment" class="Str"("Val(Sgnl)"="" ("Value (Signaling)")) -> ()  [unwired: 2 in, 2 out]
      n208 = Get Date/Time String(want seconds? (F)=TRUE) -> (date string=w359:string, time string=w357:string)  [unwired: 2 in]
      n209 = Concatenate Strings(w359, w356, w357, w356, "Add comment") -> (w355:string)
      n210 = feedback #8() -> (w354:string[])  [unwired: 1 in]
      n211 = Build Array (concatenate)(w354, w355) -> (w353:string[])
      n212 = feedback-in #8(w353) -> ()
      n213 = Write to Text File(file (use dialog)=w352, text=w353) -> ()  [unwired: 2 in, 3 out]
    }
    n214 = call "Header Names 4.vi"("Dynamic Data"=w43) -> ("Signals Out"=w44:dynamicdata)  [unwired: 10 in]
    n215 = call "Write To Measurement File"("Signals"=w44, "Enable"="OK Button 2", "Filename"=w86) -> ()  [unwired: 14 in, 3 out]
    "Boolean" <- "OK Button 2"
  }
